vi "WriteReadN.vi"(1 "Handle":i32, 2 "Axis":u32, 3 "Delay (ms)":u32=10, 4 "Move to (um)":dbl min=0.0 max=200.0 step=0.1 format="%.4f") -> (0 "Current Position (um)":dbl format="%.2f")   [LabVIEW 2012]
uses:
  Madlib.dll
panel:
  # "This example commands the nanopositioner to move to a position,\nwaits a period of time for the nanopositioner to arrive at the position,\nand then reads the position of the  nanopositioner."
  # "X = 1\nY = 2\nZ = 3"
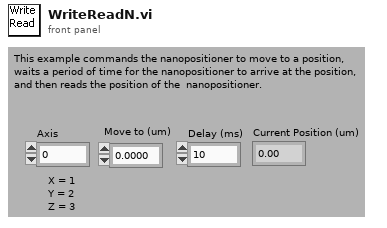
[diagram p1: front panel]
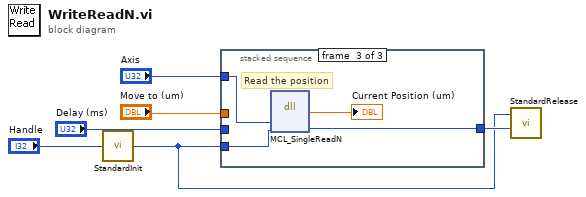
[diagram p0: block diagram]
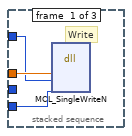
[diagram p2: hidden frame]
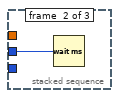
[diagram p3: hidden frame]
diagram:
  n1 = call "StandardInit.vi"("Incoming Handle"="Handle") -> ("Outgoing Handle"=w1:i32)
  n2 = stacked-sequence {
    tunnel: "Move to (um)" -> [w9 _ _]
    tunnel: "Delay (ms)" -> [_ w10 _]
    tunnel: "Axis" -> [w7 _ w14]
    tunnel: w1 -> [w8 _ w13]
    tunnel: [_ _ w11] -> w2
    frame #0 {
      # "Write"
      n3 = dll-call lib="C:/Users/Labview/Desktop/SRR/Madlib_x64/Labview Examples/MADLib.dll" fn="MCL_SingleWriteN"("position"=w9, "axis"=w7, "handle"=w8) -> ()  [unwired: 7 in, 2 out]
    }
    frame #1 {
      n4 = Wait (ms)(milliseconds to wait=w10) -> ()  [unwired: 1 out]
    }
    frame #2 {
      # "Read the position"
      n5 = dll-call lib="C:/Users/Labview/Desktop/SRR/Madlib_x64/Labview Examples/MADLib.dll" fn="MCL_SingleReadN"("axis"=w14, "handle"=w13) -> (→"Current Position (um)":dbl, "handle"=w11:i32)  [unwired: 4 in, 2 out]
    }
  }
  n6 = call "StandardRelease.vi"("Outgoing Handle"=w2, "Incoming Handle"=w1) -> ()  [unwired: 1 in]
